vi "Wait on Promise.vi"(8 "error in (no error)":errorcluster, 9 "timeout in ms (-1)":i32=-1, 11 "Future in":refnum<class "Promise.lvclass">) -> (0 "error out":errorcluster, 1 "timed out?":bool, 2 "Value":variant, 3 "Future out":refnum<class "Promise.lvclass">)   [LabVIEW 2017, in "Promise.lvlib" / "Promise.lvclass"]
uses:
  Promise.lvclass
  Promise.lvclass/Promise.ctl
  Rejected Promise/Rejected Promise.lvclass
  Rejected Promise/Rejected Promise.lvclass/Rejected Promise.ctl
  Rejected Promise/Read Reason.vi
  <vilib>/Utility/error.llb/Error Cluster From Error Code.vi
  <vilib>/ErrorRing/Error Ring.xnode
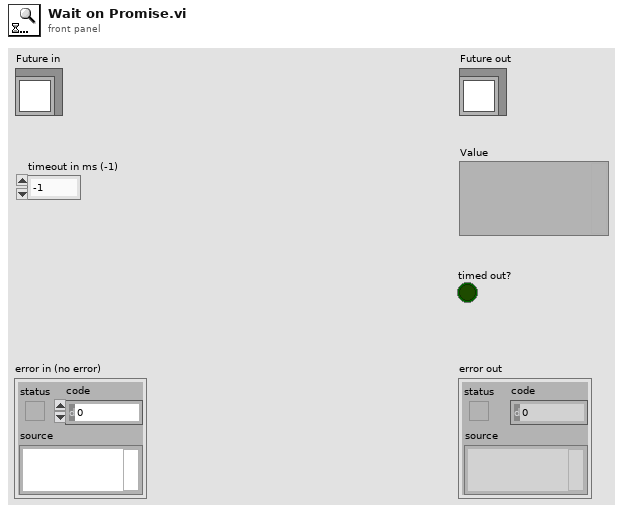
[diagram p1: front panel]
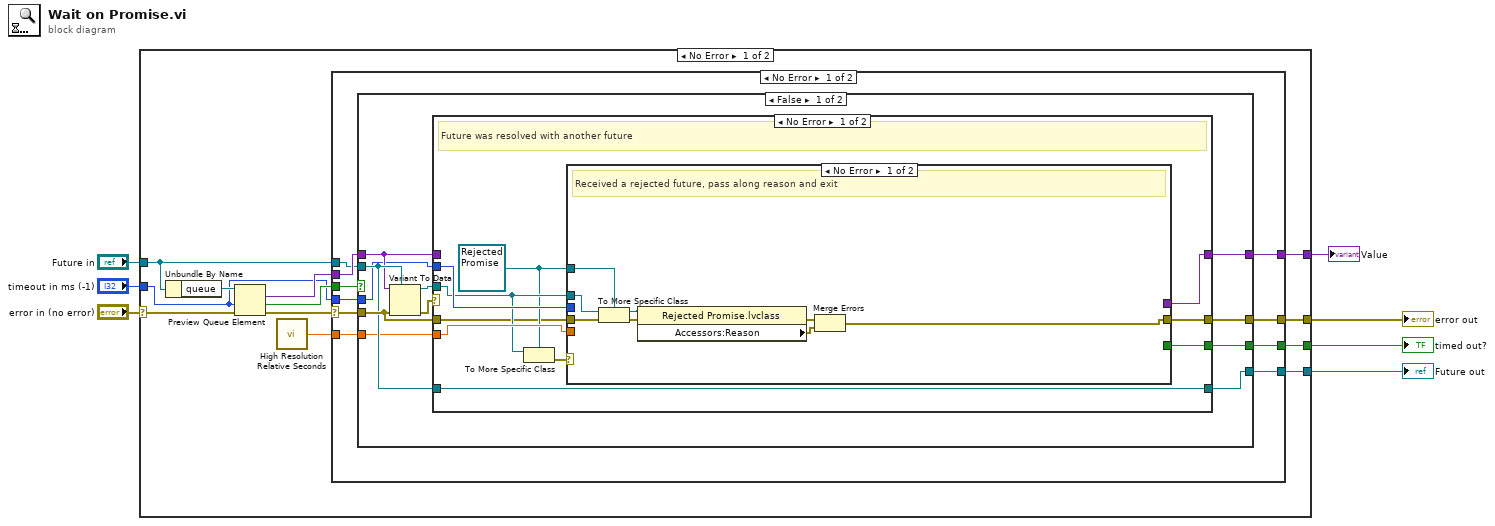
[diagram p0: block diagram]
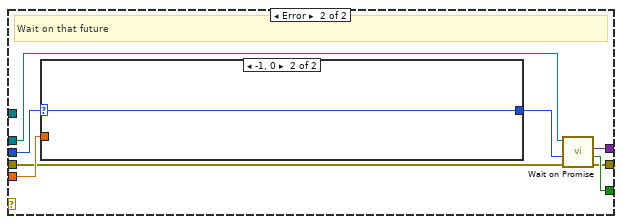
[diagram p2: hidden frame]
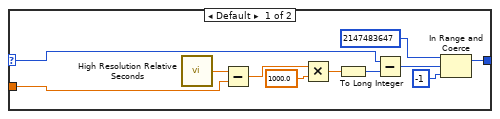
[diagram p3: hidden frame]
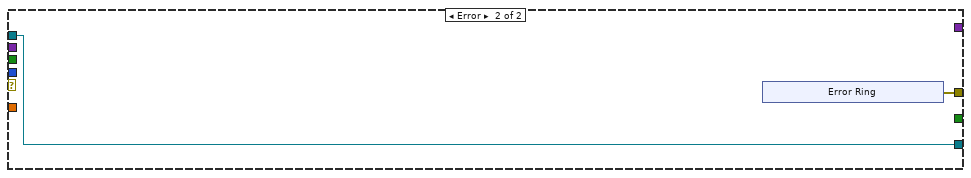
[diagram p6: hidden frame]
diagram:
  n1 = case shown="No Error" "error in (no error)" {
    selector: "error in (no error)" -> [w18 w94]
    tunnel: [w13 w94] -> w2
    tunnel: [w10 w93] -> w5
    tunnel: "Future in" -> [w11 w93]
    tunnel: [w12 _] -> w4
    tunnel: [w14 _] -> w3
    tunnel: "timeout in ms (-1)" -> [w9 _]
    frame No Error {
      n2 = Unbundle By Name(w11) -> ("queue"=w19:refnum<queue>)
      n3 = Preview Queue Element(queue=w19, timeout in ms (-1)=w9, error in (no error)=w18) -> (element=w16:variant, timed out?=w17:bool, error out=w15:errorcluster)  [unwired: 1 out]
      n4 = call <vilib>:"High Resolution Relative Seconds.vi"() -> ("relative seconds"=w8:dbl)
      n5 = case shown="No Error" w15 {
        selector: w15 -> [w27 _]
        tunnel: w17 -> [w29 _]
        tunnel: w16 -> [w28 _]
        tunnel: [w26 _] -> w14
        tunnel: [w25 w87] -> w13
        tunnel: [w24 _] -> w12
        tunnel: w11 -> [w23 w86]
        tunnel: [w22 w86] -> w10
        tunnel: w9 -> [w21 _]
        tunnel: w8 -> [w20 _]
        frame No Error {
          n6 = case shown="False" w29 {
            selector: w29 -> [_ w83]
            tunnel: w28 -> [w32 w85]
            tunnel: w27 -> [w39 w84]
            tunnel: [w40 w85] -> w26
            tunnel: [w38 w84] -> w25
            tunnel: [w36 w83] -> w24
            tunnel: w23 -> [w35 w82]
            tunnel: [w34 w82] -> w22
            tunnel: w20 -> [w31 _]
            tunnel: w21 -> [w30 _]
            frame False {
              n7 = Variant To Data(error in=w39, type=w35, Variant=w32) -> (data=w33:refnum<class "Promise.lvclass">, error out=w37:errorcluster)
              n8 = case shown="No Error" w37 {
                tunnel: [w50 w79] -> w40
                tunnel: w39 -> [w41 w81]
                tunnel: [w48 w81] -> w38
                tunnel: [w49 _] -> w36
                tunnel: w35 -> [w47 w80]
                tunnel: [w47 w80] -> w34
                tunnel: w33 -> [w43 _]
                tunnel: w32 -> [_ w79]
                tunnel: w31 -> [w45 _]
                tunnel: w30 -> [w46 _]
                frame No Error {
                  w42 = refnum<class "Rejected Promise.lvclass"> refnum ("Future.lvlib:Rejected Future.lvclass")
                  # "Future was resolved with another future"
                  n9 = To More Specific Class(target class=w42, reference=w43) -> (error out=w44:errorcluster)  [unwired: 1 in, 1 out]
                  n10 = case shown="No Error" w44 {
                    tunnel: [_ w66] -> w50
                    tunnel: [_ w65] -> w49
                    tunnel: [w51 w64] -> w48
                    tunnel: w46 -> [_ w63]
                    tunnel: w45 -> [_ w62]
                    tunnel: w43 -> [w58 w60]
                    tunnel: w42 -> [w57 _]
                    tunnel: w41 -> [w55 w59]
                    frame No Error {
                      # "Received a rejected future, pass along reason and exit"
                      n11 = To More Specific Class(target class=w57, reference=w58, error in=w55) -> (specific class reference=w56:refnum<class "Rejected Promise.lvclass">, error out=w54:errorcluster)
                      n12 = property class="Rejected Promise.lvclass"(reference=w56, error in=w54) -> (error out=w53:errorcluster, "Accessors:Reason"=w52:errorcluster)  [unwired: 1 out]
                      n13 = Merge Errors(w53, w52) -> (w51:errorcluster)
                    }
                    frame Error {
                      # "Wait on that future"
                      n14 = case shown="-1, 0" w63 {
                        selector: w63 -> [w77 w78]
                        tunnel: w62 -> [w75 _]
                        tunnel: [w69 w78] -> w61
                        frame Default {
                          n15 = call <vilib>:"High Resolution Relative Seconds.vi"() -> ("relative seconds"=w76:dbl)
                          n16 = Subtract(x=w76, y=w75) -> (x-y=w74:dbl)
                          n17 = Multiply(x=w74, y=1000.0 ("x")) -> (x*y=w72:dbl)
                          n18 = To Long Integer(number=w72) -> (32bit integer=w71:i32)
                          n19 = Subtract(x=w77, y=w71) -> (x-y=w70:i32)
                          n20 = In Range and Coerce(upper limit=2147483647, x=w70, lower limit=-1) -> (coerced(x)=w69:i32)  [unwired: 1 out]
                        }
                        frame -1, 0 {
                        }
                      }
                      n21 = call "Wait on Promise.vi"("error in (no error)"=w59, "timeout in ms (-1)"=w61, "Future in"=w60) -> ("error out"=w64:errorcluster, "timed out?"=w65:bool, "Value"=w66:variant)  [unwired: 5 in, 1 out]
                    }
                  }
                }
                frame Error {
                  # "Just a normal value, pass it along"
                }
              }
            }
            frame True {
            }
          }
        }
        frame Error {
          n22 = xnode "Error Ring"() -> ("error out"=w87:errorcluster)
        }
      }
    }
    frame Error {
    }
  }
  "error out" <- w2
  "Future out" <- w5
  "Value" <- w3
  "timed out?" <- w4
